vi "MG3700 Baseband Reference Clock Source.vi"(4 "Error in (no error)":errorcluster, 5 "Trigger (Internal)":T1, 6 "Set/Get (Set)":T2, 7 "VISA In":refnum<visa-resource-name>) -> (0 "Error out":errorcluster, 1 "Error code":i32, 2 "Trigeer out":T1, 3 "VISA Out":refnum<visa-resource-name>)   [LabVIEW 2015]
doc: "Function: Selects a baseband reference clock (external or internal)."
uses:
  MG3700A/Controls/Set_Get.ctl
  MG3700A/Controls/Int_Ext.ctl
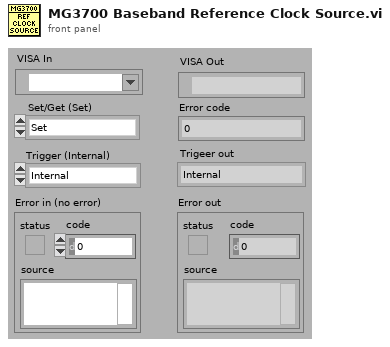
[diagram p1: front panel]
types:
  T1 = typedef "Int_Ext.ctl" = enum16{"Internal", "External"}
  T2 = typedef "Set_Get.ctl" = enum16{"Set", "Get"}
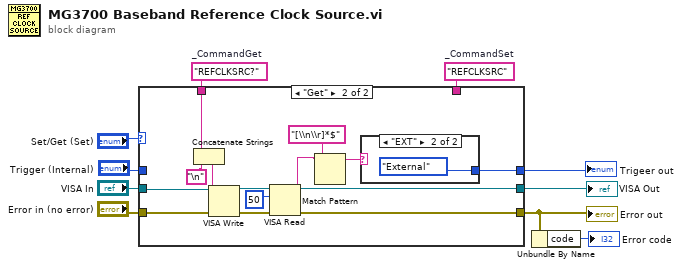
[diagram p0: block diagram]
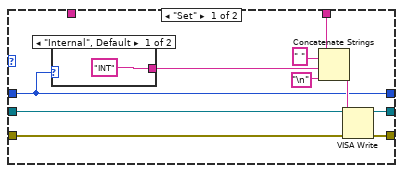
[diagram p2: hidden frame]
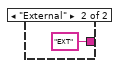
[diagram p3: hidden frame]
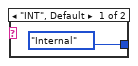
[diagram p4: hidden frame]
diagram:
  w3 = "REFCLKSRC?"  # _CommandGet
  w4 = "REFCLKSRC"  # _CommandSet
  n1 = case shown="\"Get\"" "Set/Get (Set)" {
    tunnel: "VISA In" -> [w20 w36]
    tunnel: [w19 w30] -> w9
    tunnel: [w18 w31] -> w7
    tunnel: "Error in (no error)" -> [w17 w35]
    tunnel: "Trigger (Internal)" -> [w13 _]
    tunnel: [w13 w29] -> w2
    tunnel: w4 -> [w11 _]
    tunnel: w3 -> [_ w26]
    frame "Set" {
      n2 = case shown="\"Internal\", Default" w13 {
        tunnel: ["INT" "EXT"] -> w12
        frame "Internal", Default {
        }
        frame "External" {
        }
      }
      n3 = Concatenate Strings(w11, " " ("Substring"), w12, "\n") -> (w15:string)
      n4 = VISA Write(VISA resource name=w20, write buffer=w15, error in (no error)=w17) -> (VISA resource name out=w18:refnum<visa-resource-name>, error out=w19:errorcluster)  [unwired: 1 out]
    }
    frame "Get" {
      n5 = Concatenate Strings(w26, "\n") -> (w27:string)
      n6 = VISA Write(VISA resource name=w36, write buffer=w27, error in (no error)=w35) -> (VISA resource name out=w34:refnum<visa-resource-name>, error out=w33:errorcluster)  [unwired: 1 out]
      n7 = VISA Read(VISA resource name=w34, byte count=u32 50 ("byte count (0)"), error in (no error)=w33) -> (VISA resource name out=w31:refnum<visa-resource-name>, read buffer=w24:string, error out=w30:errorcluster)  [unwired: 1 out]
      n8 = Match Pattern(string=w24, regular expression="[\\n\\r]*$") -> (before substring=w25:string)  [unwired: 1 in, 3 out]
      n9 = case shown="\"EXT\"" w25 {
        tunnel: [Int_Ext."Internal" ("Trigeer out 2") Int_Ext."External" ("Trigeer out 2")] -> w29
        frame "INT", Default {
        }
        frame "EXT" {
        }
      }
    }
  }
  "VISA Out" <- w7
  "Error out" <- w9
  "Trigeer out" <- w2
  n10 = Unbundle By Name(w9) -> ("code"=→"Error code":i32)
